vi "modulated_temperature_simulation.vi"() -> ()   [LabVIEW 2025]
panel:
  out "Verlauf":T1(graph)
  in  "stop":bool
  out "Warnung Durchschnittstemperatur":bool
  out "Warnung Tagestemperatur":bool
  in  "Schwelle Durchschnittstemperatur (°C)":dbl(slide) scale=-10.0..45.0
  in  "Schwelle Tagestemperatur (°C)":dbl(slide) scale=-10.0..45.0
  in  "Rauschfaktor (°C)":dbl(slide) scale=0.0..20.0
  in  "Schwankungen (°C)":dbl(slide) scale=0.0..20.0
  in  "Basiswert (°C)":dbl(slide) scale=-10.0..45.0
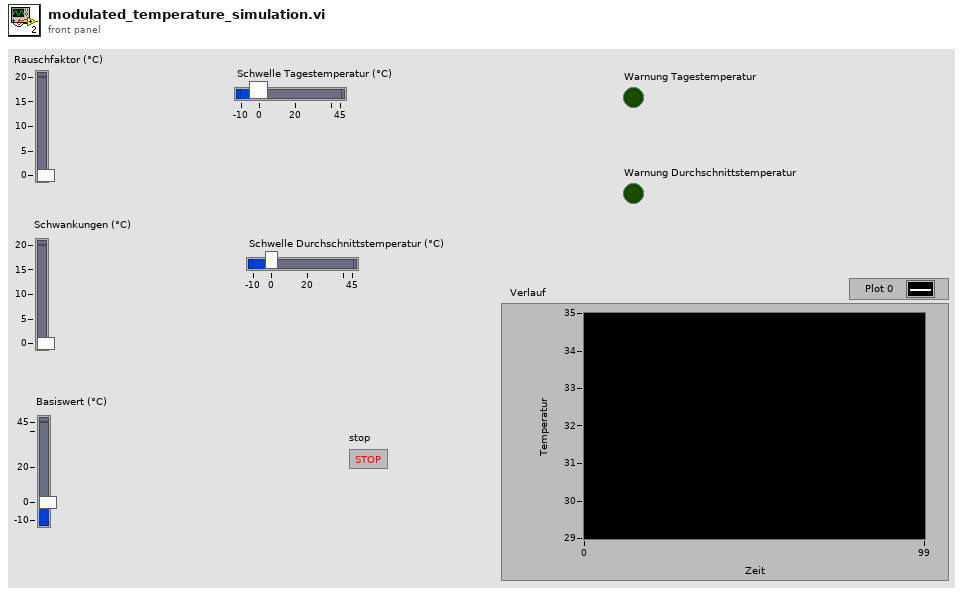
[diagram p1: front panel]
types:
  T1 = cluster{"Tagestemperatur (°C)":dbl, "Durchschnittstemperatur (°C)":dbl, "Schwelle Tagestemperatur (°C)":dbl, "Schwelle Durchschnittstemperatur (°C)":dbl}
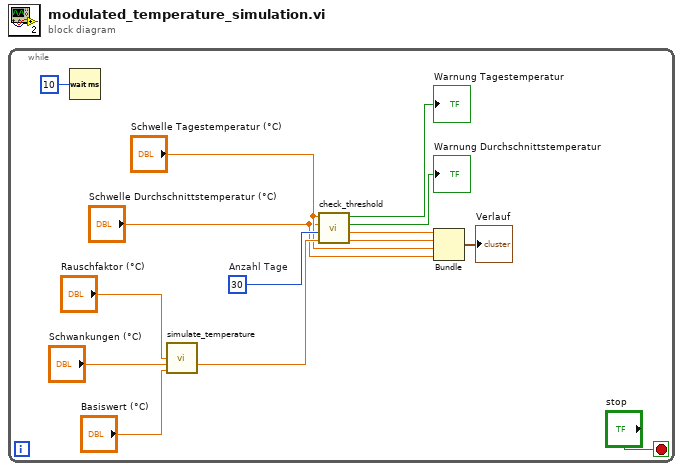
[diagram p0: block diagram]
diagram:
  n1 = while {
    stop <- "stop" stop-if-true
    w11 = 30  # Anzahl Tage
    n2 = Wait (ms)(milliseconds to wait=u32 10) -> ()  [unwired: 1 out]
    n3 = call "simulate_temperature.vi"("Rauschfaktor"="Rauschfaktor (°C)", "Schwankungen"="Schwankungen (°C)", "Basiswert"="Basiswert (°C)") -> ("Temperaturwert (°C)"=w10:dbl)  [unwired: 12 in]
    n4 = call "check_threshold.vi"("Schwelle Tagestemperatur (°C)"="Schwelle Tagestemperatur (°C)", "Schwelle Durchschnittstemperatur (°C)"="Schwelle Durchschnittstemperatur (°C)", "Anzahl Tage"=w11, "Temperature"=w10) -> ("Warnung Tagestemperatur"=→"Warnung Tagestemperatur":bool, "Warnung Durchschnittstemperatur"=→"Warnung Durchschnittstemperatur":bool, "Tagestemperatur (°C)"=w7:dbl, "Durchschnittstemperatur (°C)"=w6:dbl)  [unwired: 3 in]
    n5 = Bundle("Tagestemperatur (°C)"=w7, "Durchschnittstemperatur (°C)"=w6, "Schwelle Tagestemperatur (°C)"="Schwelle Tagestemperatur (°C)", "Schwelle Durchschnittstemperatur (°C)"="Schwelle Durchschnittstemperatur (°C)") -> (→"Verlauf":T1)  [unwired: 1 in]
  }
